vi "SubVI_CalculateRange.vi"(8 "XScale.Minimum":dbl, 9 "XScale.Maximum":dbl, 10 "File End Time":dbl, 11 "File Start Time":dbl) -> (3 "Range":cluster{dbl, dbl})   [LabVIEW 2011]
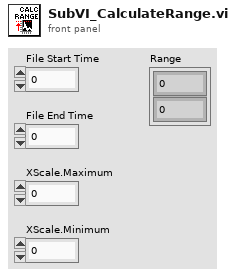
[diagram p1: front panel]
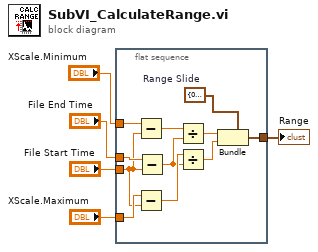
[diagram p0: block diagram]
diagram:
  n1 = flat-sequence {
    tunnel: [w15] -> w1
    tunnel: "XScale.Maximum" -> [w10]
    tunnel: "XScale.Minimum" -> [w14]
    tunnel: "File Start Time" -> [w9]
    tunnel: "File End Time" -> [w13]
    frame #0 {
      w16 = cluster{dbl, dbl} {0.44603381014304294, 0.5370611183355006}  # Range Slide
      n2 = Subtract(x=w14, y=w9) -> (x-y=w11:dbl)
      n3 = Subtract(x=w10, y=w9) -> (x-y=w8:dbl)
      n4 = Subtract(x=w13, y=w9) -> (x-y=w7:dbl)
      n5 = Divide(x=w11, y=w7) -> (x/y=w12:dbl)
      n6 = Divide(x=w8, y=w7) -> (x/y=w6:dbl)
      n7 = Bundle(cluster=w16, w12, w6) -> (w15:cluster{dbl, dbl})
    }
  }
  "Range" <- w1
